vi "Create.vi"   [LabVIEW 2021, in "Field_RnD_Services_LIBSSH2_Toolkit.lvlib" / "Listener.lvclass"]
doc: "Creates a new Listener object that represents a libssh2lv shared library Listener struct. This VI must be called, or executed, before using any other Listener-related VIs. This VI allocates memory within the libssh2lv shared library that must be explicitly deallocated, or freed, at the end of the application using the <B>Destroy</B> VI to avoid memory leaks or running Out-of-Memory (OOM) on a resource contrained system.\n\nA Listener object represents a callback that is executed when various SSH-related events occur."
uses:
  220524-VNA RP FLAT.llb/Listener.lvclass
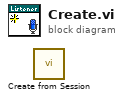
[diagram p0: block diagram]
diagram:
  n1 = call "Create from Session.vi"() -> ()  [unwired: 10 in, 2 out]
